vi "Configure Dialog.vi"(8 "Error In":errorcluster, 11 "Reset Device Msg in":refnum<class "Reset Device Msg.lvclass">) -> (0 "Error Out":errorcluster, 2 "OK?":bool, 3 "Reset Device Msg out":refnum<class "Reset Device Msg.lvclass">)   [LabVIEW 2014, in "CS++DeviceActor.lvlib" / "Reset Device Msg.lvclass"]
doc: "This overrides of this dynamic dispatch VI open the frontpanel to set derived message attributes."
uses:
  Reset Device Msg.lvclass
panel:
  in  "OK":bool
  in  "Cancel":bool
  # "Do you really want to reset the device?"
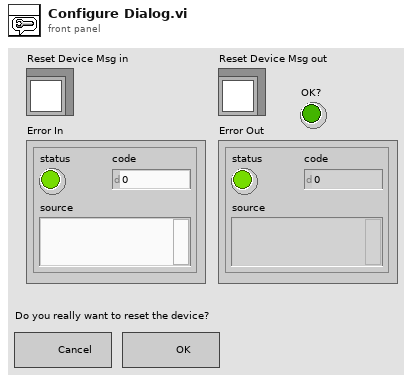
[diagram p1: front panel]
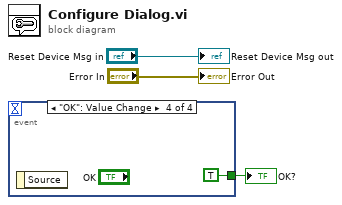
[diagram p0: block diagram]
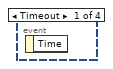
[diagram p2: hidden frame]
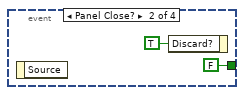
[diagram p3: hidden frame]
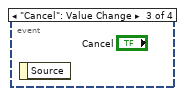
[diagram p4: hidden frame]
diagram:
  n1 = event shown="[3] \"OK\": Value Change" {
    selector: _ -> [_ _ _ _]
    dyn-events: _ -> [_ _ _ _]
    timeout: _ -> [_ _ _ _]
    tunnel: [_ FALSE _ TRUE] -> w1
    event Timeout {
      n2 = event-data() -> ()  [unwired: 1 in, 1 out]
    }
    event Panel Close? {
      n3 = event-data() -> ()  [unwired: 1 in, 1 out]
      n4 = event-data("Discard?"=TRUE) -> ()  [unwired: 1 in, 1 out]
    }
    event "Cancel": Value Change {
      n5 = event-data() -> ()  [unwired: 1 in, 1 out]
    }
    event "OK": Value Change {
      n6 = event-data() -> ()  [unwired: 1 in, 1 out]
    }
  }
  "OK?" <- w1
  "Error Out" <- "Error In"
  "Reset Device Msg out" <- "Reset Device Msg in"
